vi "Acquisition Message Loop.vi"(8 "error in (no error)":errorcluster, 9 "Data Queue":T1, 10 "Data Notifier":T2, 11 "Message Queues":T3) -> (0 "error out":errorcluster)   [LabVIEW 2015, in "Acquisition.lvlib"]
doc: "Message loop for handling messages pertaining to the acquisition of data from the hardware."
uses:
  Acquisition.lvlib
  Support VIs/Message Queue/All Message Queues.ctl
  Support VIs/Message Queue/Message Cluster.ctl
  controls/Data notifier.ctl
  Generic data packet.ctl
  My Graphs/Gps Map Graph coordinates.ctl
  controls/Data queue.ctl
  Hardware Configuration.ctl
  Acquisition State.ctl
  Support VIs/Message Queue/Enqueue Message (Single).vi
  <vilib>/Utility/error.llb/Error Cluster From Error Code.vi
  <vilib>/ErrorRing/Error Ring.xnode
  Support VIs/Message Queue/Message Queue.lvlib
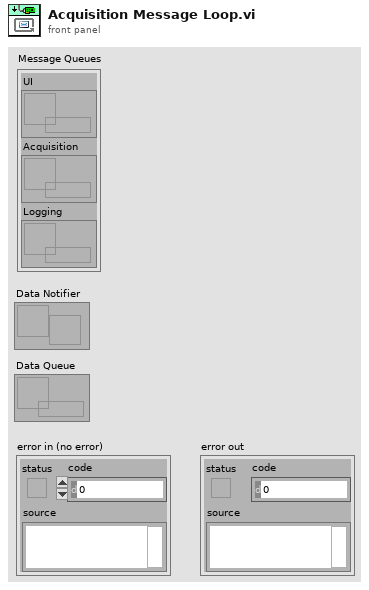
[diagram p1: front panel]
types:
  T1 = typedef "Data queue.ctl" = refnum<queue>
  T2 = typedef "Data notifier.ctl" = refnum<notifier>
  T3 = typedef "Message Queue.lvlib/All Message Queues.ctl" = cluster{"UI":refnum<queue>, "Acquisition":refnum<queue>, "Logging":refnum<queue>}
  T4 = typedef "Acquisition.lvlib/Hardware Configuration.ctl" = cluster{"Data source":enum16{"Serial port", "Simulated data", "Web page JSON"}, "Connection info":cluster{"VISA resource name":refnum<visa-resource-name>, "Baud rate":u32, "data bits":u16, "stop bits":u16, "parity (0:none)":enum16{"None", "Odd", "Even", "Mark", "Space"}, "flow control (0:none)":u16, "timeout (10sec)":u32, "termination char\n(0xA = '\\n' = LF) ":u8, "Enable Termination\nChar (T)":bool}, "Protocol info":cluster{"Temination char":u8, "Escape char":u8}, "Internet server":cluster{"Web page telemetry":string, "Web page gps":string}, "Data format":enum16{"IDRA data", "XAM data"}}
  T5 = typedef "Acquisition.lvlib/Acquisition State.ctl" = enum16{"Idle", "Acquiring"}
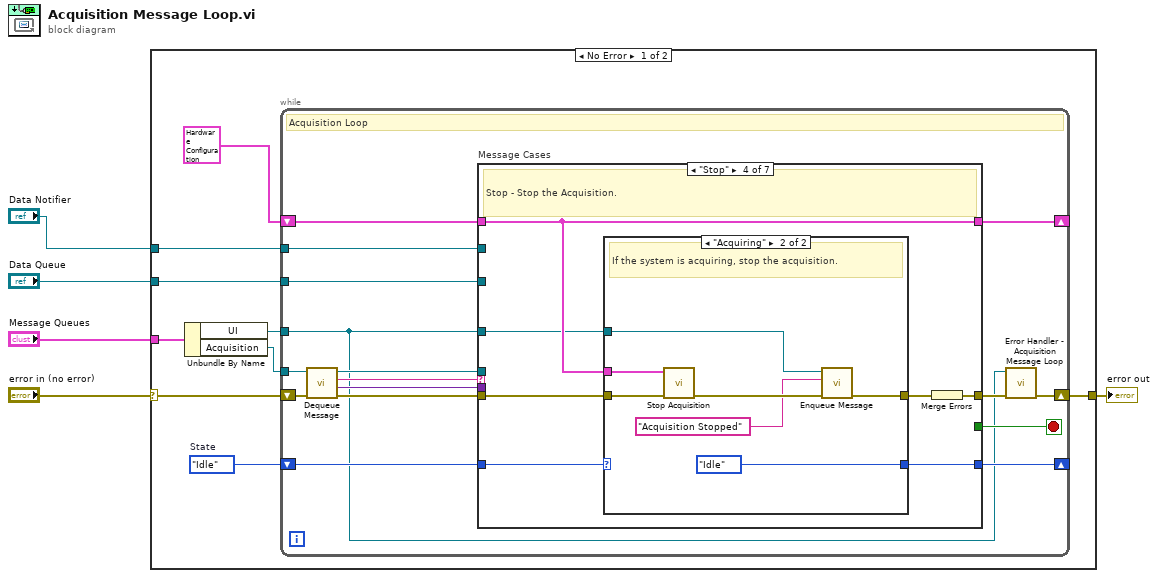
[diagram p0: block diagram]
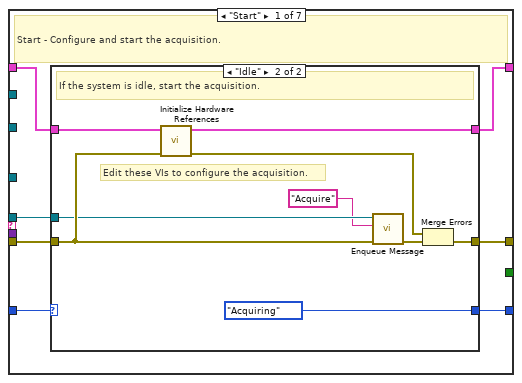
[diagram p2: hidden frame]
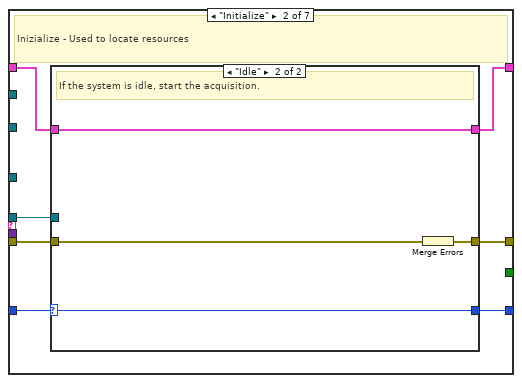
[diagram p4: hidden frame]
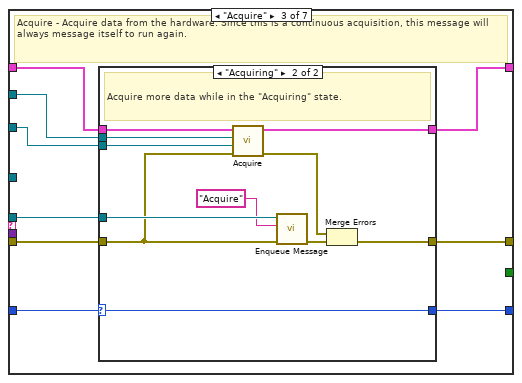
[diagram p6: hidden frame]
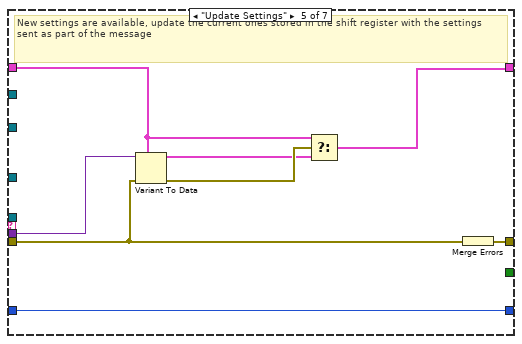
[diagram p9: hidden frame]
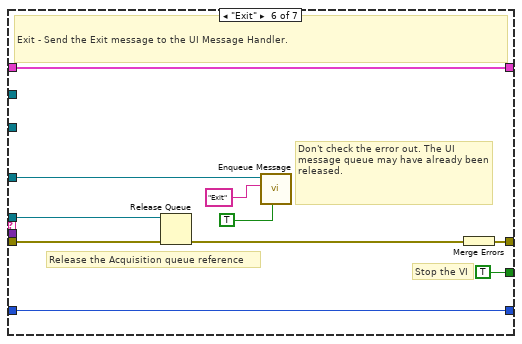
[diagram p10: hidden frame]
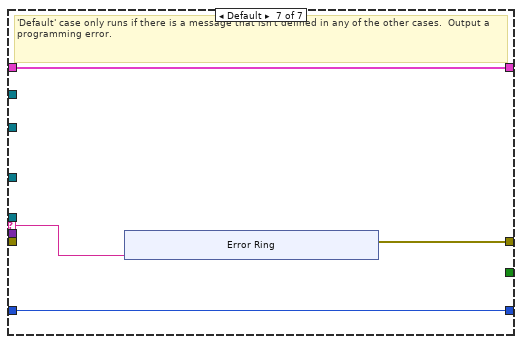
[diagram p11: hidden frame]
diagram:
  n1 = case shown="No Error" "error in (no error)" {
    selector: "error in (no error)" -> [w10 w132]
    tunnel: "Message Queues" -> [w14 _]
    tunnel: [w12 w132] -> w4
    tunnel: "Data Notifier" -> [w8 _]
    tunnel: "Data Queue" -> [w7 _]
    frame No Error {
      w6 = Acquisition_State."Idle"  # State
      n2 = Unbundle By Name(w14) -> ("UI"=w9:refnum<queue>, "Acquisition"=w13:refnum<queue>)
      n3 = while {
        tunnel: w13 -> [w23]
        shift-right: [w29] -> _
        shift-left: T4 {"Data source"=enum."Serial port", "Connection info"={"VISA resource name"="", "Baud rate"=0, "data bits"=0, "stop bits"=0, "parity (0:none)"=enum."None", "flow control (0:none)"=0, "timeout (10sec)"=0, "termination char\n(0xA = '\\n' = LF) "=0, "Enable Termination\nChar (T)"=FALSE}, "Protocol info"={"Temination char"=255, "Escape char"=254}, "Internet server"={"Web page telemetry"="", "Web page gps"=""}, "Data format"=enum."IDRA data"} ("Data Cluster") -> [w30]
        shift-right: [w18] -> w12
        shift-left: w10 -> [w27]
        tunnel: w9 -> [w15]
        tunnel: w8 -> [w22]
        tunnel: w7 -> [w21]
        shift-right: [w19] -> _
        shift-left: w6 -> [w20]
        stop <- w28 stop-if-true
        # "Acquisition Loop"
        n4 = call "Dequeue Message.vi"("error in (no error)"=w27, "Message Queue"=w23) -> ("error out"=w26:errorcluster, "Message Data"=w24:variant, "Message"=w25:string, "dup Message Queue"=w16:refnum<queue>)  [unwired: 6 in]
        n5 = case "Message Cases" shown="\"Stop\"" w25 {
          selector: w25 -> [_ _ _ _ _ _ w121]
          tunnel: w16 -> [w34 w53 w71 _ _ w112 _]
          tunnel: w26 -> [w35 w54 w70 w92 w104 w116 _]
          tunnel: [w37 w56 w72 w93 w110 w119 w122] -> w17
          tunnel: w30 -> [w36 w55 w68 w90 w106 w118 w124]
          tunnel: [w33 w52 w69 w90 w105 w118 w124] -> w29
          tunnel: [_ _ _ _ _ TRUE _] -> w28
          tunnel: w24 -> [_ _ _ _ w109 _ _]
          tunnel: w15 -> [_ _ _ w87 _ w117 _]
          tunnel: w22 -> [_ _ w67 _ _ _ _]
          tunnel: w21 -> [_ _ w66 _ _ _ _]
          tunnel: w20 -> [w31 w50 w64 w89 w103 w111 w123]
          tunnel: [w32 w51 w65 w88 w103 w111 w123] -> w19
          frame "Start" {
            # "Start - Configure and start the acquisition."
            n6 = case shown="\"Idle\"" w31 {
              selector: w31 -> [w38 _]
              tunnel: [w39 w49] -> w37
              tunnel: w36 -> [w40 w48]
              tunnel: w35 -> [w39 w47]
              tunnel: w34 -> [_ w45]
              tunnel: [w40 w41] -> w33
              tunnel: [w38 Acquisition_State."Acquiring" ("Acquisition State")] -> w32
              frame "Acquiring" {
                # "The system is already acquiring. Ignore the \"Start\" message."
              }
              frame "Idle" {
                # "Edit these VIs to configure the acquisition."
                # "If the system is idle, start the acquisition."
                n7 = call "Initialize Hardware References.vi"("error in"=w47, "Hardware Resources in"=w48) -> ("error out"=w42:errorcluster, "Hardware Resources out"=w41:T4)  [unwired: 8 in]
                n8 = call-poly "Enqueue Message.vi"("error in (no error)"=w47, "Message"="Acquire", "Message Queue"=w45) -> ("error out"=w46:errorcluster)  [unwired: 7 in, 1 out]
                n9 = Merge Errors(w42, w46) -> (w49:errorcluster)
              }
            }
          }
          frame "Initialize" {
            # "Inizialize - Used to locate resources"
            n10 = case shown="\"Idle\"" w50 {
              selector: w50 -> [w57 w60]
              tunnel: [w58 w63] -> w56
              tunnel: w55 -> [w59 w62]
              tunnel: w54 -> [w58 w61]
              tunnel: w53 -> [_ _]
              tunnel: [w59 w62] -> w52
              tunnel: [w57 w60] -> w51
              frame "Acquiring" {
                # "The system is already acquiring. Ignore the \"Inizielize\" message."
              }
              frame "Idle" {
                # "If the system is idle, start the acquisition."
                n11 = Merge Errors(w61) -> (w63:errorcluster)
              }
            }
          }
          frame "Acquire" {
            # "Acquire - Acquire data from the hardware. Since this is a continuous acquisition, this message will always message itself to run again."
            n12 = case shown="\"Acquiring\"" w64 {
              selector: w64 -> [w73 w77]
              tunnel: [w74 w86] -> w72
              tunnel: w71 -> [_ w84]
              tunnel: w70 -> [w74 w76]
              tunnel: [w75 w82] -> w69
              tunnel: w68 -> [w75 w81]
              tunnel: w67 -> [_ w79]
              tunnel: w66 -> [_ w78]
              tunnel: [w73 w77] -> w65
              frame "Idle" {
                # "Ignore \"Acquire\" messages when the acquisition is idle."
              }
              frame "Acquiring" {
                # "Acquire more data while in the \"Acquiring\" state."
                n13 = call "Acquire.vi"("error in (no error)"=w76, "Data Queue"=w78, "Data Notifier"=w79, "Hardware Resources in"=w81) -> ("error out"=w83:errorcluster, "Hardware Resources out"=w82:T4)  [unwired: 6 in]
                n14 = call-poly "Enqueue Message.vi"("error in (no error)"=w76, "Message"="Acquire", "Message Queue"=w84) -> ("error out"=w85:errorcluster)  [unwired: 7 in, 1 out]
                n15 = Merge Errors(w83, w85) -> (w86:errorcluster)
              }
            }
          }
          frame "Stop" {
            # "Stop - Stop the Acquisition."
            n16 = case shown="\"Acquiring\"" w89 {
              selector: w89 -> [w94 _]
              tunnel: w92 -> [w95 w102]
              tunnel: [w95 w98] -> w91
              tunnel: w90 -> [_ w100]
              tunnel: [w94 Acquisition_State."Idle" ("State")] -> w88
              tunnel: w87 -> [_ w97]
              frame "Idle" {
                # "The system is already idle. Ignore the \"Stop\" message."
              }
              frame "Acquiring" {
                # "If the system is acquiring, stop the acquisition."
                n17 = call "Stop Acquisition.vi"("error in (no error)"=w102, "Hardware Resources in"=w100) -> ("error out"=w101:errorcluster)  [unwired: 9 in]
                n18 = call-poly "Enqueue Message.vi"("error in (no error)"=w101, "Message"="Acquisition Stopped", "Message Queue"=w97) -> ("error out"=w98:errorcluster)  [unwired: 7 in, 1 out]
              }
            }
            n19 = Merge Errors(w91) -> (w93:errorcluster)
          }
          frame "Update Settings" {
            # "New settings are available, update the current ones stored in the shift register with the settings sent as part of the message"
            n20 = Variant To Data(error in=w104, type=w106, Variant=w109) -> (data=w107:T4, error out=w108:errorcluster)
            n21 = Select(t=w106, s=w108, f=w107) -> (s? t:f=w105:T4)
            n22 = Merge Errors(w104) -> (w110:errorcluster)
          }
          frame "Exit" {
            # "Don't check the error out. The UI message queue may have already been released."
            # "Release the Acquisition queue reference"
            # "Stop the VI"
            # "Exit - Send the Exit message to the UI Message Handler."
            n23 = Release Queue(queue=w112, error in (no error)=w116) -> (error out=w113:errorcluster)  [unwired: 1 in, 2 out]
            n24 = call-poly "Enqueue Message.vi"("Priority Message? (F)"=TRUE, "Message"="Exit", "Message Queue"=w117) -> ()  [unwired: 7 in, 2 out]
            n25 = Merge Errors(w113) -> (w119:errorcluster)
          }
          frame Default {
            # "'Default' case only runs if there is a message that isn't defined in any of the other cases.  Output a programming error."
            n26 = xnode "Error Ring"("parameter 0"=w121) -> ("error out"=w122:errorcluster)
          }
        }
        n27 = call "Error Handler - Acquisition Message Loop.vi"("error in (no error)"=w17, "Message Queue"=w15) -> ("dup error in"=w18:errorcluster)  [unwired: 8 in, 1 out]
      }
    }
    frame Error {
    }
  }
  "error out" <- w4
